vi "Open Engine Simulation Toolkit System Definition.vi"(8 "error in (no error)":errorcluster, 10 "System Definition Path":path, 11 "Current VI in":refnum<vi>) -> (0 "error out":errorcluster, 2 "Engine Simulation Toolkit NodeID":u64, 3 "SystemDefinition":refnum<k24>)   [LabVIEW 2020, in "Mutation Test Case.lvclass"]
uses:
  Mutation Test Case.lvclass
  NationalInstruments.VeriStand.SystemDefinitionAPI
  Shared/Constants and GUIDs.vi
  <userlib>/_OpenG.lib/file/file.llb/Append Path to Root if Relative - Scalar__ogtk.vi
  <vilib>/NI/VeriStand Custom Device Testing Tools/VeriStandTestUtilities/VeriStandTestUtilities.lvlib
  Shared/Engine Simulation Toolkit Shared.lvlib
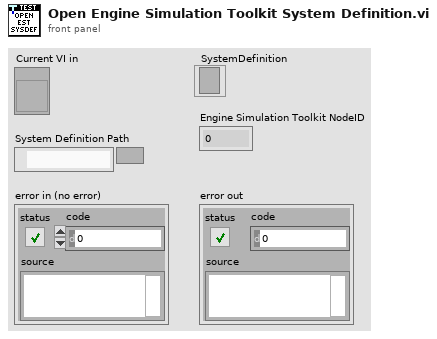
[diagram p1: front panel]
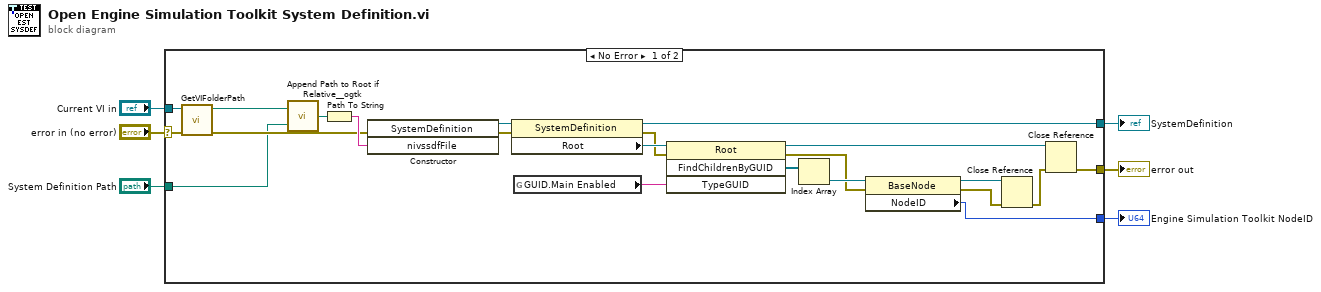
[diagram p0: block diagram]
diagram:
  n1 = case shown="No Error" "error in (no error)" {
    selector: "error in (no error)" -> [w14 w29]
    tunnel: [w28 _] -> w6
    tunnel: [w27 w29] -> w5
    tunnel: [w20 _] -> w4
    tunnel: "System Definition Path" -> [w9 _]
    tunnel: "Current VI in" -> [w7 _]
    frame No Error {
      n2 = call <vilib>:"GetVIFolderPath.vi"("error in (no error)"=w14, "VI Reference in"=w7) -> ("error out"=w10:errorcluster, "VI Folder Path out"=w8:path)  [unwired: 8 in]
      n3 = call-poly <userlib>:"Append Path to Root if Relative__ogtk.vi"("Absolute or Relative Path"=w9, "Root Path"=w8) -> ("Absolute or Appended Path"=w22:path)
      n4 = Path To String(path=w22) -> (string=w12:string)
      n5 = constructor class="SystemDefinition"(error in=w10, "nivssdfFile"=w12) -> (reference out=w13:refnum<k24>, error out=w11:errorcluster)  [unwired: 2 in, 2 out]
      n6 = property class="SystemDefinition"(reference=w13, error in=w11) -> (reference out=w28:refnum<k24>, error out=w15:errorcluster, "Root"=w16:refnum<k24>)
      n7 = global read "Constants and GUIDs.vi" "GUID.Main Enabled"() -> (w17:string)
      n8 = invoke class="Root" method="FindChildrenByGUID"(reference=w16, error in=w15, "TypeGUID"=w17) -> (reference out=w26:refnum<k24>, error out=w19:errorcluster, "FindChildrenByGUID"=w18:refnum<k24>[])  [unwired: 1 in, 1 out]
      n9 = Index Array(array=w18) -> (element=w21:refnum<k24>)  [unwired: 1 in]
      n10 = property class="BaseNode"(reference=w21, error in=w19) -> (reference out=w24:refnum<k24>, error out=w23:errorcluster, "NodeID"=w20:u64)
      n11 = Close Reference(reference=w24, error in (no error)=w23) -> (error out=w25:errorcluster)
      n12 = Close Reference(reference=w26, error in (no error)=w25) -> (error out=w27:errorcluster)
    }
    frame Error {
    }
  }
  "SystemDefinition" <- w6
  "error out" <- w5
  "Engine Simulation Toolkit NodeID" <- w4
